vi "Constant flow for an amount of time.vi"() -> ()   [LabVIEW 2018]
uses:
  <vilib>/Instr/_visa.llb/VISA Configure Serial Port (Instr).vi
  <instrlib>/SF-10/SF-10.lvlib
panel:
  out "Elapsed Time (s)":dbl
  in  "stop":bool
  in  "Mode (0: FLOW)":u16(ring) items=["FLOW", "RAMP"]
  in  "VISA resource name":refnum<visa-resource-name>
  in  "Flowrate (1 ml/min)":dbl=1.0
  in  "Time Target (1 min)":dbl=1.0 caption="Time Target (s)"
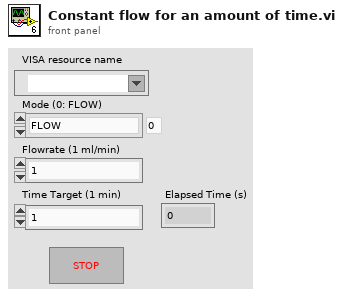
[diagram p1: front panel]
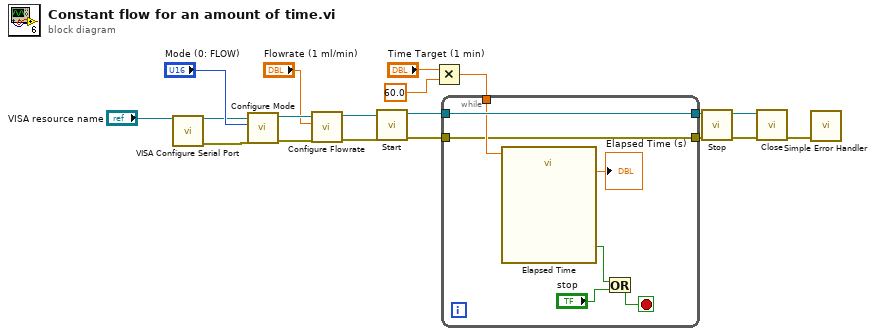
[diagram p0: block diagram]
diagram:
  n1 = call-poly "VISA Configure Serial Port"("VISA resource name"="VISA resource name") -> ("VISA resource name out"=w2:refnum<visa-resource-name>, "error out"=w1:errorcluster)  [unwired: 13 in]
  n2 = call <instrlib>:"Configure Mode.vi"("error in (no error)"=w1, "Mode (0: FLOW)"="Mode (0: FLOW)", "VISA resource name"=w2) -> ("error out"=w17:errorcluster, "VISA resource name out"=w19:refnum<visa-resource-name>)  [unwired: 6 in]
  n3 = call <instrlib>:"Configure Flowrate.vi"("error in (no error)"=w17, "Flowrate (1 ml/min)"="Flowrate (1 ml/min)", "VISA resource name"=w19) -> ("error out"=w16:errorcluster, "VISA resource name out"=w18:refnum<visa-resource-name>)  [unwired: 7 in]
  n4 = call <instrlib>:"Start.vi"("error in (no error)"=w16, "VISA resource name"=w18) -> ("error out"=w12:errorcluster, "VISA resource name out"=w14:refnum<visa-resource-name>)  [unwired: 8 in]
  n5 = Multiply(x="Time Target (1 min)", y=60.0) -> (x*y=w4:dbl)
  n6 = while {
    tunnel: w14 -> [w26]
    tunnel: [w26] -> w13
    tunnel: w4 -> [w25]
    tunnel: [w24] -> w11
    tunnel: w12 -> [w24]
    stop <- w22 stop-if-true
    n7 = call "Elapsed Time"("Time Target (s)"=w25) -> ("Elapsed Time (s)"=→"Elapsed Time (s)":dbl, "Time has Elapsed"=w21:bool)  [unwired: 11 in, 6 out]
    n8 = Or(x=w21, y="stop") -> (x .or. y?=w22:bool)
  }
  n9 = call <instrlib>:"Stop.vi"("error in (no error)"=w11, "VISA resource name"=w13) -> ("error out"=w10:errorcluster, "VISA resource name out"=w9:refnum<visa-resource-name>)  [unwired: 8 in]
  n10 = call <instrlib>:"Close.vi"("error in (no error)"=w10, "VISA resource name"=w9) -> ("error out"=w8:errorcluster)  [unwired: 9 in]
  n11 = call <vilib>:"Simple Error Handler.vi"("error in (no error)"=w8) -> ()  [unwired: 4 in, 5 out]
